vi "Write 1Ch 1Samp (DBL).vi"(5 "timestamp":timestamp, 7 "index_channel":u32, 8 "error in":errorcluster, 9 "data":dbl, 10 "channel":u32, 11 "writer":u64) -> (0 "error out":errorcluster, 3 "writer out":u64)   [LabVIEW 2026, in "synnax_clib.lvlib"]
uses:
  synnax_clib.lvlib
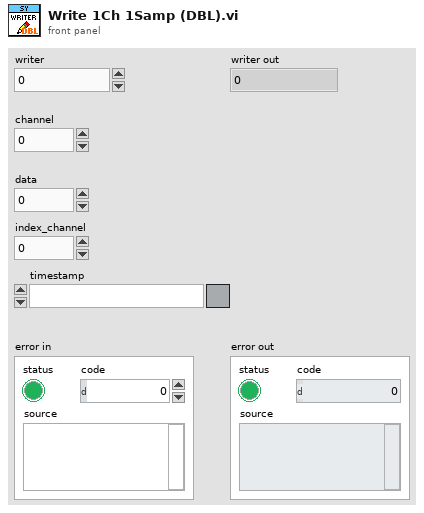
[diagram p1: front panel]
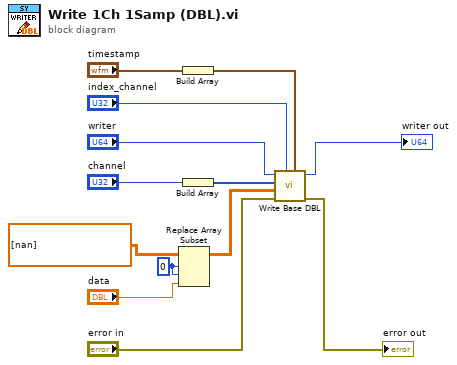
[diagram p0: block diagram]
diagram:
  w3 = 0
  n1 = Replace Array Subset(array=dbl[][] [nan], new element="data", index (row)=w3, index (col)=w3) -> (w1:dbl[][])
  n2 = Build Array("timestamp") -> (w5:timestamp[])
  n3 = Build Array("channel") -> (w8:u32[])
  n4 = call "Write Base DBL.vi"("timestamps"=w5, "index_channel"="index_channel", "error in"="error in", "data"=w1, "channels"=w8, "writer"="writer") -> ("error out"=→"error out":errorcluster, "writer out"=→"writer out":u64)  [unwired: 4 in]
